vi "DataLog Interpolate Log.vi"(0 "tag log directory":path, 5 "tag config":T2 {"logging parameters" format="%.2e"; "precision" items=["0", "1", "2", "3", "4", "5", "6", "7", "8", "9", "10", "11", "12", "13", "14", "15", "16", "17"]; "limit delay" format="%.2e"; "deadband" format="%.2e"}, 7 "times":dbl[](array[numeric]) format="%<%H:%M:%S%2u\n%Y/%m/%d>T", 11 "error in (no error)":errorcluster) -> (4 "dup tag log directory":path, 6 "value type":T1, 8 "interpolated values":dbl[](array[numeric]), 15 "error out":errorcluster)   [LabVIEW 2012]
doc: "Interpolate the point values in a tag log at the specified times. When the tag is of \"sample\" temporal type, the values of the two points adjacent to each specified time are linearly interpolated in case of a number tag, or, in case of a string tag, an error is returned. When the tag is of \"set&hold\" temporal type, the value of the last point prior to each specified time is used: such tags hold their value until changed. In case of a string tag you'll have to use the returned offset values to read the string values from the log. When the tag is of \"event\" temporal type, an error is returned since such tags have values that are defined only at the time of the event.\n\nNote that this VI tries to read the timerange covered by the specified times from the tag log before commencing with interpolation. This fails when the timerange contains more than \"max points\" points. In such an event, the specified times are divided in increasingly smaller chunks until the reads succeed. In this eventuality, it helps performance when the specified times increase or decrease monotonically."
uses:
  typedefs/clusters/t_DataLog Tag Config.ctl
  typedefs/t_DataLog Temporal Types.ctl
  typedefs/t_DataLog Value Types.ctl
  typedefs/t_DataLog Numerical Format.ctl
  typedefs/t_DataLog Logging Algorithms.ctl
  private/glb_DataLog Runtime Parameterisation.vi
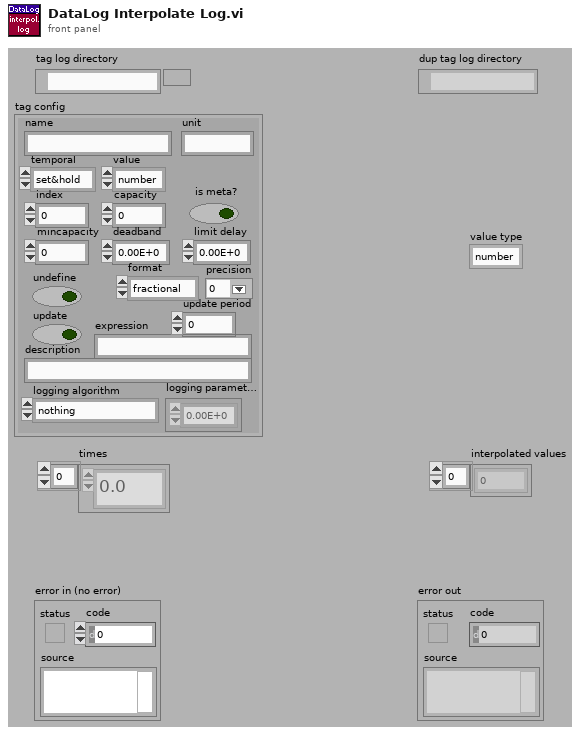
[diagram p1: front panel]
types:
  T1 = typedef "t_DataLog Value Types.ctl" = enum16{"number", "string"}
  T2 = typedef "t_DataLog Tag Config.ctl" = cluster{"name":string, "unit":string, "temporal":T3, "value":T1, "index":i32, "capacity":i32, "is meta?":bool, "mincapacity":i32, "deadband":dbl, "limit delay":dbl, "format":T4, "precision":u8, "undefine":bool, "update":bool, "update period":u16, "expression":string, "description":string, "logging algorithm":T5, "logging parameters":dbl[]}
  T3 = typedef "t_DataLog Temporal Types.ctl" = enum16{"set&hold", "sample", "event"}
  T4 = typedef "t_DataLog Numerical Format.ctl" = enum8{"fractional", "exponential", "engineering"}
  T5 = typedef "t_DataLog Logging Algorithms.ctl" = enum16{"nothing", "changes", "everything", "every Nth", "time threshold", "value threshold + prior", "t or v threshold", "t or v threshold + prior"}
  T6 = typedef "t_DataLog Point.ctl" = cluster{"time":dbl, "value":dbl}
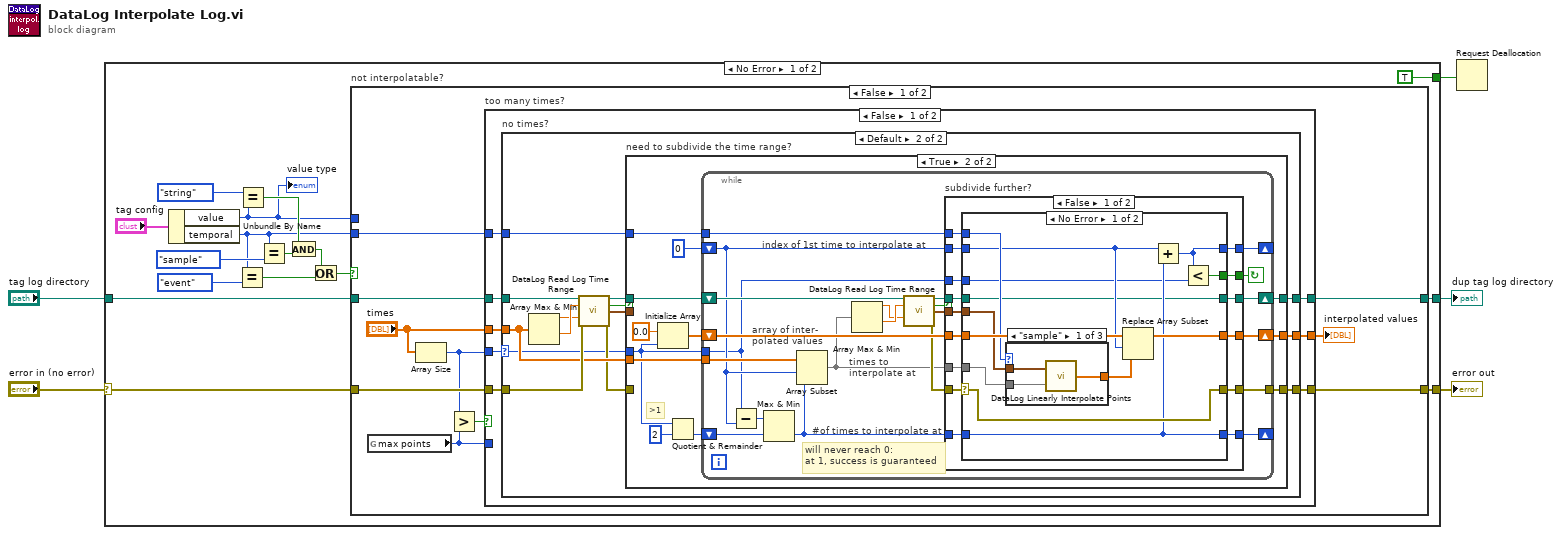
[diagram p0: block diagram]
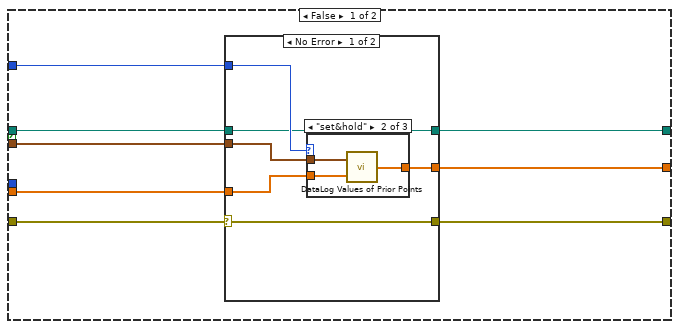
[diagram p3: hidden frame]
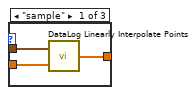
[diagram p4: hidden frame]
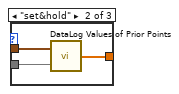
[diagram p7: hidden frame]
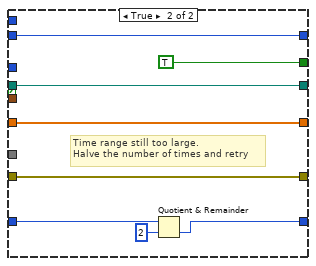
[diagram p10: hidden frame]
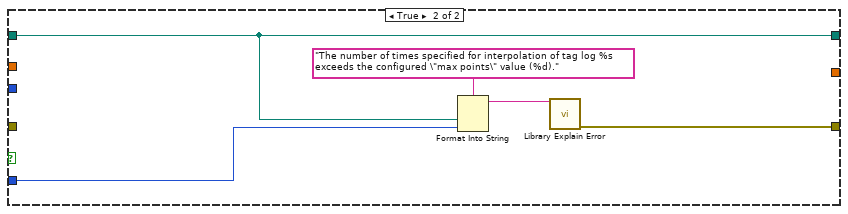
[diagram p11: hidden frame]
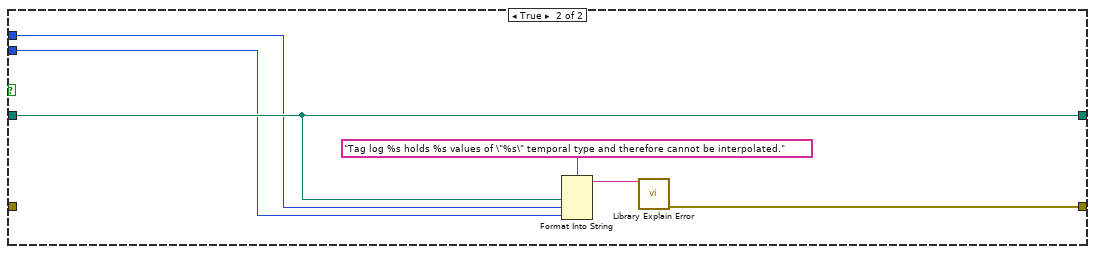
[diagram p12: hidden frame]
diagram:
  n1 = case shown="No Error" "error in (no error)" {
    selector: "error in (no error)" -> [w21 w170]
    tunnel: [w18 w170] -> w5
    tunnel: "tag log directory" -> [w20 w169]
    tunnel: [w19 w169] -> w2
    tunnel: [TRUE _] -> w1
    frame No Error {
      n2 = Unbundle By Name("tag config") -> ("value"=w8:T1, "temporal"=w11:T3)
      "value type" <- w8
      n3 = Equal?(x=w11, y=t_DataLog_Temporal_Types."event" ("temporal")) -> (x = y?=w9:bool)
      n4 = Equal?(x=t_DataLog_Value_Types."string" ("value type"), y=w8) -> (x = y?=w12:bool)
      n5 = Equal?(x=w11, y=t_DataLog_Temporal_Types."sample" ("temporal")) -> (x = y?=w13:bool)
      n6 = And(x=w12, y=w13) -> (x .and. y?=w10:bool)
      n7 = Or(x=w10, y=w9) -> (x .or. y?=w7:bool)
      n8 = case "not interpolatable?" shown="False" w7 {
        tunnel: w21 -> [w31 _]
        tunnel: w20 -> [w30 w166]
        tunnel: [w29 w166] -> w19
        tunnel: [w28 w168] -> w18
        tunnel: w11 -> [w25 w163]
        tunnel: w8 -> [_ w164]
        frame False {
          n9 = global read "glb_DataLog Runtime Parameterisation.vi" "max points"() -> (w24:i32)
          n10 = Array Size(array="times") -> (size(s)=w23:i32)
          n11 = Greater?(x=w23, y=w24) -> (0:w26:bool)
          n12 = case "too many times?" shown="False" w26 {
            tunnel: w31 -> [w39 _]
            tunnel: w30 -> [w38 w158]
            tunnel: [w35 w158] -> w29
            tunnel: [w34 w160] -> w28
            tunnel: "times" -> [w37 _]
            tunnel: w24 -> [_ w159]
            tunnel: w25 -> [w36 _]
            tunnel: w23 -> [w32 _]
            tunnel: [w33 _] -> w22
            frame False {
              n13 = case "no times?" shown="Default" w32 {
                selector: w32 -> [_ w42]
                tunnel: w39 -> [w41 w55]
                tunnel: w38 -> [w40 w52]
                tunnel: w37 -> [_ w50]
                tunnel: w36 -> [_ w49]
                tunnel: [w40 w47] -> w35
                tunnel: [w41 w46] -> w34
                tunnel: [_ w43] -> w33
                frame 0 {
                  # "no times => no interpolated values"
                }
                frame Default {
                  n14 = Array Max & Min(array=w50) -> (max value=w53:dbl, min value=w54:dbl)  [unwired: 2 out]
                  n15 = call "DataLog Read Log Time Range.vi"("tag log directory"=w52, "begin of range"=w54, "end of range"=w53, "error in (no error)"=w55) -> ("dup tag log directory"=w48:path, "too many points?"=w44:bool, "time range of points"=w51:T6[], "error out"=w45:errorcluster)  [unwired: 8 in]
                  n16 = case "need to subdivide the time range?" shown="True" w44 {
                    tunnel: [w62 w85] -> w43
                    tunnel: w50 -> [w61 w84]
                    tunnel: w49 -> [w60 w78]
                    tunnel: w48 -> [w57 w88]
                    tunnel: [w56 w89] -> w47
                    tunnel: [w58 w79] -> w46
                    tunnel: w45 -> [w59 _]
                    tunnel: w51 -> [w63 _]
                    tunnel: w42 -> [_ w80]
                    frame False {
                      n17 = case shown="No Error" w59 {
                        selector: w59 -> [w65 w77]
                        tunnel: w63 -> [w69 _]
                        tunnel: [w68 _] -> w62
                        tunnel: w61 -> [w67 _]
                        tunnel: w60 -> [w66 _]
                        tunnel: [w65 w77] -> w58
                        tunnel: w57 -> [w64 w76]
                        tunnel: [w64 w76] -> w56
                        frame No Error {
                          n18 = case shown="\"set&hold\"" w66 {
                            tunnel: w69 -> [w72 w75 _]
                            tunnel: [w71 w74 _] -> w68
                            tunnel: w67 -> [w70 w73 _]
                            frame "sample" {
                              n19 = call "DataLog Linearly Interpolate Points.vi"("times"=w70, "points"=w72) -> ("interpolated values"=w71:dbl[])
                            }
                            frame "set&hold" {
                              n20 = call "DataLog Values of Prior Points.vi"("times"=w73, "points"=w75) -> ("prior values"=w74:dbl[])
                            }
                            frame "event" {
                            }
                          }
                        }
                        frame Error {
                        }
                      }
                    }
                    frame True {
                      # ">1"
                      n21 = Initialize Array(0.0, w80) -> (w86:dbl[])
                      n22 = Quotient & Remainder(x=w80, y=2) -> (floor(x/y)=w83:i32)  [unwired: 1 out]
                      n23 = while {
                        shift-right: [w111] -> w89
                        shift-left: w88 -> [w101]
                        shift-right: [w107] -> w85
                        shift-left: w86 -> [w109]
                        tunnel: w84 -> [w102]
                        shift-right: [w110] -> _
                        shift-left: w83 -> [w106]
                        shift-right: [w108] -> _
                        shift-left: 0 ("y") -> [w95]
                        tunnel: w80 -> [w90]
                        tunnel: [w104] -> w79
                        tunnel: w78 -> [w91]
                        stop <- w94 continue-if-true
                        # "will never reach 0:\nat 1, success is guaranteed"
                        # "array of inter-\npolated values"
                        # "times to\ninterpolate at"
                        # "index of 1st time to interpolate at"
                        # "#of times to interpolate at"
                        n24 = Subtract(x=w90, y=w95) -> (x-y=w105:i32)
                        n25 = Max & Min(x=w105, y=w106) -> (min(x,y)=w103:i32)  [unwired: 1 out]
                        n26 = Array Subset(array=w102, index=w95, length=w103) -> (w93:dbl[])
                        n27 = Array Max & Min(array=w93) -> (max value=w99:dbl, min value=w100:dbl)  [unwired: 2 out]
                        n28 = call "DataLog Read Log Time Range.vi"("tag log directory"=w101, "begin of range"=w100, "end of range"=w99) -> ("dup tag log directory"=w97:path, "too many points?"=w98:bool, "time range of points"=w92:T6[], "error out"=w96:errorcluster)  [unwired: 9 in]
                        n29 = case "subdivide further?" shown="False" w98 {
                          tunnel: [w126 w152] -> w111
                          tunnel: [w125 w154] -> w110
                          tunnel: w109 -> [w124 w151]
                          tunnel: [w123 w153] -> w108
                          tunnel: [w122 w151] -> w107
                          tunnel: [w121 w150] -> w104
                          tunnel: w103 -> [w120 w155]
                          tunnel: w97 -> [w119 w152]
                          tunnel: w96 -> [w118 w150]
                          tunnel: w95 -> [w117 w153]
                          tunnel: [w113 TRUE] -> w94
                          tunnel: w93 -> [w116 _]
                          tunnel: w92 -> [w115 _]
                          tunnel: w91 -> [w114 _]
                          tunnel: w90 -> [w112 _]
                          frame False {
                            n30 = case shown="No Error" w118 {
                              selector: w118 -> [w135 w147]
                              tunnel: w119 -> [w130 w149]
                              tunnel: [w130 w149] -> w126
                              tunnel: w120 -> [w131 w148]
                              tunnel: [w131 w148] -> w125
                              tunnel: [w135 w147] -> w121
                              tunnel: w124 -> [w139 _]
                              tunnel: w117 -> [w132 w146]
                              tunnel: [w128 w146] -> w123
                              tunnel: [w134 _] -> w122
                              tunnel: w116 -> [w136 _]
                              tunnel: w115 -> [w138 _]
                              tunnel: w114 -> [w137 _]
                              tunnel: [w129 _] -> w113
                              tunnel: w112 -> [w127 _]
                              frame No Error {
                                n31 = case shown="\"sample\"" w137 {
                                tunnel: w138 -> [w142 w145 _]
                                tunnel: [w141 w144 _] -> w133
                                tunnel: w136 -> [w140 w143 _]
                                frame "sample" {
                                n32 = call "DataLog Linearly Interpolate Points.vi"("times"=w140, "points"=w142) -> ("interpolated values"=w141:dbl[])
                                }
                                frame "set&hold" {
                                n33 = call "DataLog Values of Prior Points.vi"("times"=w143, "points"=w145) -> ("prior values"=w144:dbl[])
                                }
                                frame "event" {
                                }
                                }
                                n34 = Replace Array Subset(array=w139, new element=w133, index=w132) -> (w134:dbl[])
                                n35 = Add(x=w132, y=w131) -> (x+y=w128:i32)
                                n36 = Less?(x=w128, y=w127) -> (x < y?=w129:bool)
                              }
                              frame Error {
                              }
                            }
                          }
                          frame True {
                            # "Time range still too large.\nHalve the number of times and retry"
                            n37 = Quotient & Remainder(x=w155, y=2) -> (floor(x/y)=w154:i32)  [unwired: 1 out]
                          }
                        }
                      }
                    }
                  }
                }
              }
            }
            frame True {
              n38 = Format Into String(format string="The number of times specified for interpolation of tag log %s exceeds the configured \"max points\" value (%d).", w158, w159) -> (resulting string=w162:string)  [unwired: 2 in, 1 out]
              n39 = call "Library Explain Error.vi"("explanation prefix (none)"=w162) -> ("explained error"=w160:errorcluster)  [unwired: 14 in]
            }
          }
          "interpolated values" <- w22
        }
        frame True {
          n40 = Format Into String(format string="Tag log %s holds %s values of \"%s\" temporal type and therefore cannot be interpolated.", w166, w164, w163) -> (resulting string=w167:string)  [unwired: 2 in, 1 out]
          n41 = call "Library Explain Error.vi"("explanation prefix (none)"=w167) -> ("explained error"=w168:errorcluster)  [unwired: 14 in]
        }
      }
    }
    frame Error {
    }
  }
  "error out" <- w5
  "dup tag log directory" <- w2
  n42 = Request Deallocation(w1) -> ()
